vi "Missing classes on LV project.vi"(8 "error in (no error)":errorcluster, 11 "Path":path) -> (0 "error out":errorcluster, 3 "Pass":bool)   [LabVIEW 2021]
panel:
  out "Numeric":i32
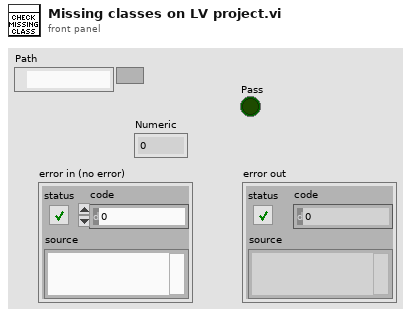
[diagram p1: front panel]
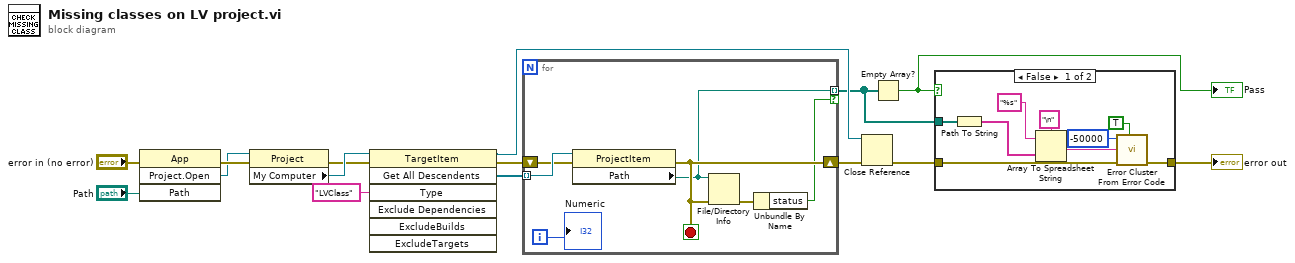
[diagram p0: block diagram]
diagram:
  n1 = invoke class="App" method="Project.Open"(error in="error in (no error)", "Path"="Path") -> (error out=w6:errorcluster, "Project:Open"=w5:refnum<vi>)  [unwired: 2 in, 2 out]
  n2 = property class="Project"(reference=w5, error in=w6) -> (error out=w12:errorcluster, "My Computer"=w15:refnum<vi>)  [unwired: 1 out]
  n3 = invoke class="TargetItem" method="Get All Descendents"(reference=w15, error in=w12, "Type"="LVClass") -> (reference out=w9:refnum<vi>, error out=w11:errorcluster, "All Descendents"=w13:refnum<vi>[])  [unwired: 4 in, 4 out]
  n4 = for {
    tunnel: w13 -> [w22] mode=indexing
    shift-right: [w19] -> w10
    shift-left: w11 -> [w21]
    tunnel: [w18] -> w2 mode=indexing if=w17
    i -> [w16]
    stop <- w19 stop-if-true
    n5 = property class="ProjectItem"(reference=w22, error in=w21) -> (error out=w19:errorcluster, "Path"=w18:path)  [unwired: 1 out]
    n6 = File/Directory Info(path=w18, error in=w19) -> (error out=w20:errorcluster)  [unwired: 6 out]
    n7 = Unbundle By Name(w20) -> ("status"=w17:bool)
    "Numeric" <- w16
  }
  n8 = Close Reference(reference=w9, error in (no error)=w10) -> (error out=w4:errorcluster)
  n9 = Empty Array?(array=w2) -> (empty?=w1:bool)
  "Pass" <- w1
  n10 = case shown="False" w1 {
    tunnel: w2 -> [w30 _]
    tunnel: [w25 w32] -> w3
    tunnel: w4 -> [w24 w32]
    frame False {
      n11 = Path To String(path=w30) -> (string=w29:string[])
      n12 = Array To Spreadsheet String(delimiter (Tab)="\n", array=w29, 3:"%s" ("format string")) -> (spreadsheet string=w26:string)
      n13 = call <vilib>:"Error Cluster From Error Code.vi"("show call chain? (False)"=TRUE, "error in (no error)"=w24, "error message (\"\")"=w26, "error code (0)"=-50000) -> ("error out"=w25:errorcluster)  [unwired: 5 in]
    }
    frame True {
    }
  }
  "error out" <- w3
